vi "InvFilter-Design.vi"(0 "Path":path, 7 "InvFilt Params":T1={"Min Frequency (Hz)"=0.0, "Max Frequency (Hz)"=0.0, "Length (points)"=301, "Sampling rate (Hz)"=0.0, "Delay (ms)"=301.0, "Linear phase"=FALSE}, 11 "error in (no error)":errorcluster) -> (4 "Interp Freq (Hz)":dbl[](array[numeric]), 6 "Magnitude (dB)":dbl[](array[numeric]), 8 "InvFilter(t)":dbl[](array[numeric]), 15 "error out":errorcluster)   [LabVIEW 2015]
uses:
  InvFilt-Params.ctl
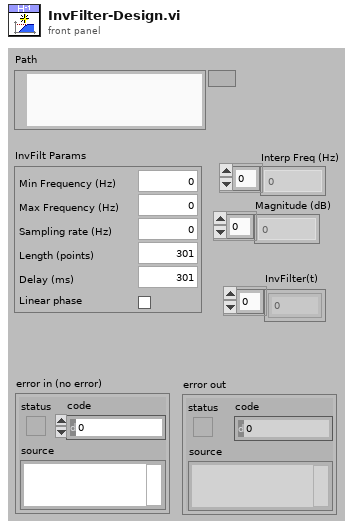
[diagram p1: front panel]
types:
  T1 = typedef "InvFilt-Params.ctl" = cluster{"Min Frequency (Hz)":dbl, "Max Frequency (Hz)":dbl, "Length (points)":i32, "Sampling rate (Hz)":dbl, "Delay (ms)":dbl, "Linear phase":bool}
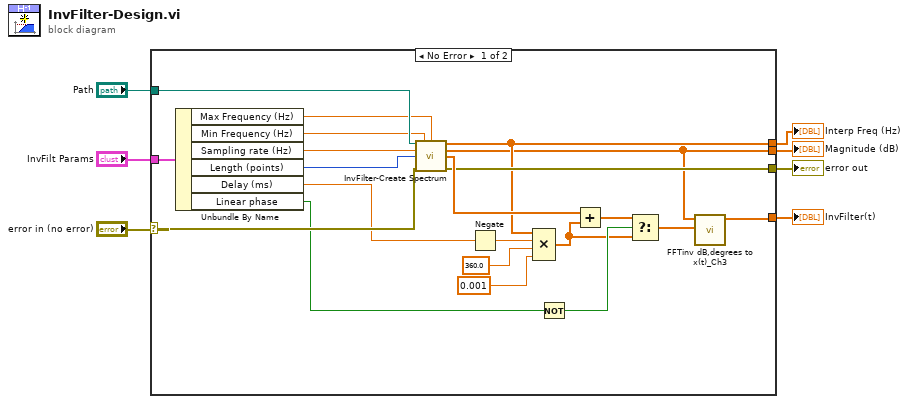
[diagram p0: block diagram]
diagram:
  n1 = case shown="No Error" "error in (no error)" {
    selector: "error in (no error)" -> [w21 w29]
    tunnel: [w20 w29] -> w6
    tunnel: "Path" -> [w24 _]
    tunnel: "InvFilt Params" -> [w23 _]
    tunnel: [w22 _] -> w3
    tunnel: [w11 _] -> w2
    tunnel: [w10 _] -> w1
    frame No Error {
      n2 = Unbundle By Name(w23) -> ("Max Frequency (Hz)"=w18:dbl, "Min Frequency (Hz)"=w17:dbl, "Sampling rate (Hz)"=w16:dbl, "Length (points)"=w9:i32, "Delay (ms)"=w19:dbl, "Linear phase"=w15:bool)
      n3 = call "InvFilter-Create Spectrum.vi"("Calibration file"=w24, "Fmin (Hz)"=w17, "Fmax (Hz)"=w18, "Fs (Hz)"=w16, "Npts"=w9, "error in (no error)"=w21) -> ("Interp Freq (Hz)"=w11:dbl[], "Magnitude (dB)"=w10:dbl[], "Phase (degrees)"=w28:dbl[], "error out"=w20:errorcluster)  [unwired: 6 in]
      n4 = Negate(x=w19) -> (-x=w27:dbl)
      n5 = Compound Arithmetic op=MULTIPLY(w11, w27, 360.0 ("Numeric"), 0.001 ("value")) -> (w12:dbl[])
      n6 = Not(x=w15) -> (.not. x?=w14:bool)
      n7 = Add(x=w28, y=w12) -> (x+y=w13:dbl[])
      n8 = Select(t=w13, s=w14, f=w12) -> (s? t:f=w8:dbl[])
      n9 = call "FFTinv dB,degrees to x(t)_Ch3.vi"("+Freq Phase of FFT (degrees)"=w8, "+Freq. Mag of FFT (rms dB)"=w10) -> ("X(t)"=w22:dbl[])  [unwired: 8 in, 1 out]
    }
    frame Error {
    }
  }
  "error out" <- w6
  "InvFilter(t)" <- w3
  "Interp Freq (Hz)" <- w2
  "Magnitude (dB)" <- w1
